vi "DAQmx Stop Task.vi"(0 "task/channels in":refnum<k21>, 11 "error in":errorcluster) -> (4 "task out":refnum<k21>, 15 "error out":errorcluster)   [LabVIEW 2013]
doc: "Stops the task and returns it to the state the task was in before the DAQmx Start Task VI ran or the DAQmx Write VI ran with the <B>autostart</B> input set to TRUE."
uses:
  nilvaiu.dll
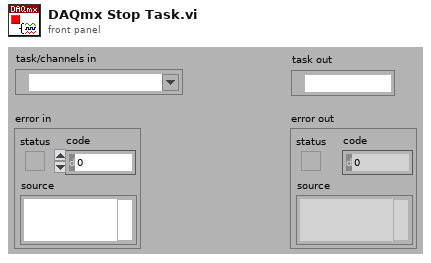
[diagram p1: front panel]
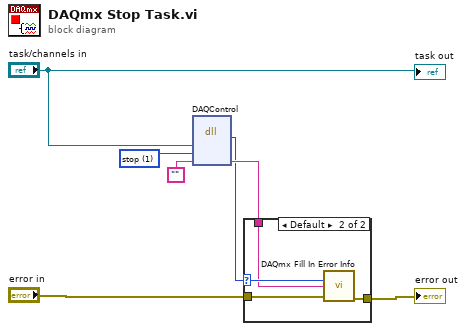
[diagram p0: block diagram]
diagram:
  w1 = u16 1 items=["stop"=1]
  n1 = dll-call lib="nilvaiu.*" fn="DAQControl"("taskID"="task/channels in", "mode"=w1, "extendedErrorInfo"="") -> (w2:i32, "extendedErrorInfo"=w3:string)  [unwired: 3 in, 4 out]
  n2 = case shown="Default" w2 {
    selector: w2 -> [_ w11]
    tunnel: [w8 w12] -> w7
    tunnel: w3 -> [_ w10]
    tunnel: "error in" -> [w8 w9]
    frame 0 {
    }
    frame Default {
      n3 = call "DAQmx Fill In Error Info.vi"("status code"=w11, "extended error info"=w10, "error in"=w9) -> ("error out"=w12:errorcluster)  [unwired: 1 in, 11 out]
    }
  }
  "error out" <- w7
  "task out" <- "task/channels in"
